vi "Read Escala Excel.vi"(8 "error in (no error)":errorcluster, 9 "Colunm":i32, 10 "row":i32, 11 "NI_report in":refnum<class "NI_report.lvclass">) -> (0 "error out":errorcluster, 2 "data":dbl, 3 "NI_report Out":refnum<class "NI_report.lvclass">)   [LabVIEW 2015]
uses:
  <vilib>/Utility/NIReport.llb/NI_report.lvclass
  <vilib>/addons/_office/excel.llb/Excel Get Data (str).vi
  <vilib>/addons/_office/NI_ReportGenerationToolkit.lvlib
  <vilib>/Utility/NIReport.llb/Excel/NI_Excel.lvclass
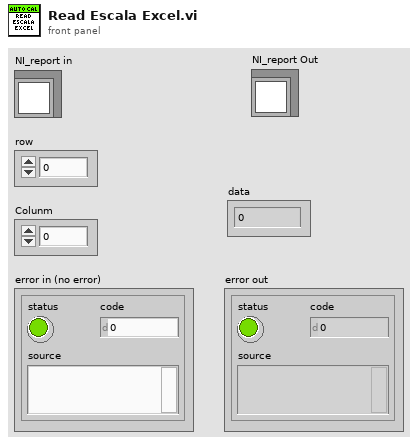
[diagram p1: front panel]
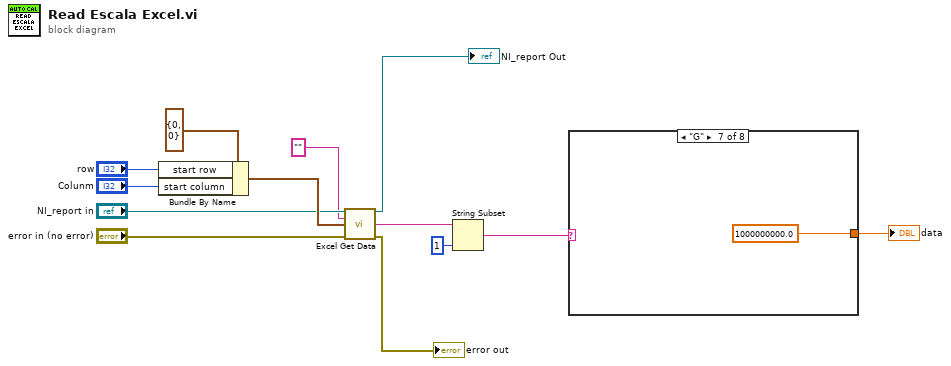
[diagram p0: block diagram]
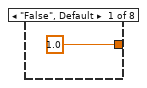
[diagram p2: hidden frame]
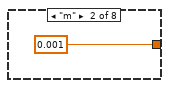
[diagram p3: hidden frame]
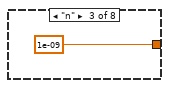
[diagram p4: hidden frame]
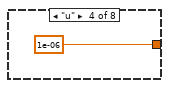
[diagram p5: hidden frame]
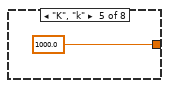
[diagram p6: hidden frame]
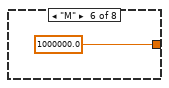
[diagram p7: hidden frame]
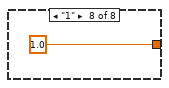
[diagram p8: hidden frame]
diagram:
  n1 = Bundle By Name(cluster=cluster{"start row":i32, "start column":i32} {"start row"=0, "start column"=0} ("start (0, 0)"), "start row"="row", "start column"="Colunm") -> (w12:cluster{"start row":i32, "start column":i32})
  n2 = call-poly <vilib>:"Excel Get Data.vi"("report in"="NI_report in", "data type"="", "start (0, 0)"=w12, "error in (no error)"="error in (no error)") -> ("report out"=→"NI_report Out":refnum<class "NI_report.lvclass">, "data"=w4:string, "error out"=→"error out":errorcluster)  [unwired: 9 in]
  n3 = String Subset(string=w4, length (rest)=1 ("length (rest)")) -> (substring=w2:string)  [unwired: 1 in]
  n4 = case shown="\"G\"" w2 {
    tunnel: [1.0 0.001 1e-09 1e-06 1000.0 1000000.0 1000000000.0 1.0] -> w1
    frame "False", Default {
    }
    frame "m" {
    }
    frame "n" {
    }
    frame "u" {
    }
    frame "K", "k" {
    }
    frame "M" {
    }
    frame "G" {
    }
    frame "1" {
    }
  }
  "data" <- w1
